vi "Read PIC SW Version.vi"(11 "Device in":refnum<class "PIC-Device.lvclass">) -> (2 "PIC SW Version":string, 3 "Device out":refnum<class "PIC-Device.lvclass">)   [LabVIEW 2020, in "PIC-Device.lvclass"]
uses:
  PIC-Device.lvclass
  PIC-Device.lvclass/PIC-Device.ctl
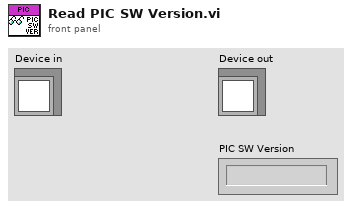
[diagram p1: front panel]
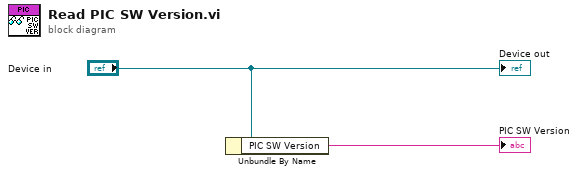
[diagram p0: block diagram]
diagram:
  n1 = Unbundle By Name("Device in") -> ("PIC SW Version"=→"PIC SW Version":string)
  "Device out" <- "Device in"
